vi "功能码解析.vi"(1 "功能码":string) -> ()   [LabVIEW 2013]
panel:
  out "24":bool[](array[boolean])
  out "23":bool[](array[boolean])
  out "22":bool[](array[boolean])
  out "21":bool[](array[boolean])
  out "20":bool[](array[boolean])
  out "19":bool[](array[boolean])
  out "18":bool[](array[boolean])
  out "17":bool[](array[boolean])
  out "16":bool[](array[boolean])
  out "15":bool[](array[boolean])
  out "14":bool[](array[boolean])
  out "13":bool[](array[boolean])
  out "12":bool[](array[boolean])
  out "主板控制类信息10":bool[](array[boolean])
  out "主板版本号11":bool[](array[boolean])
  out "主板故障阀值8":bool[](array[boolean])
  out "主板故障阀值9":bool[](array[boolean])
  out "主板项目信息7":bool[](array[boolean])
  out "主板项目信息6":bool[](array[boolean])
  out "主板项目信息5":bool[](array[boolean])
  out "主板项目信息4":bool[](array[boolean])
  out "主板项目信息3":bool[](array[boolean])
  out "主板监控2":bool[](array[boolean])
  out "主板监控预留1":bool[](array[boolean])
  # "从左到右，从高到低"
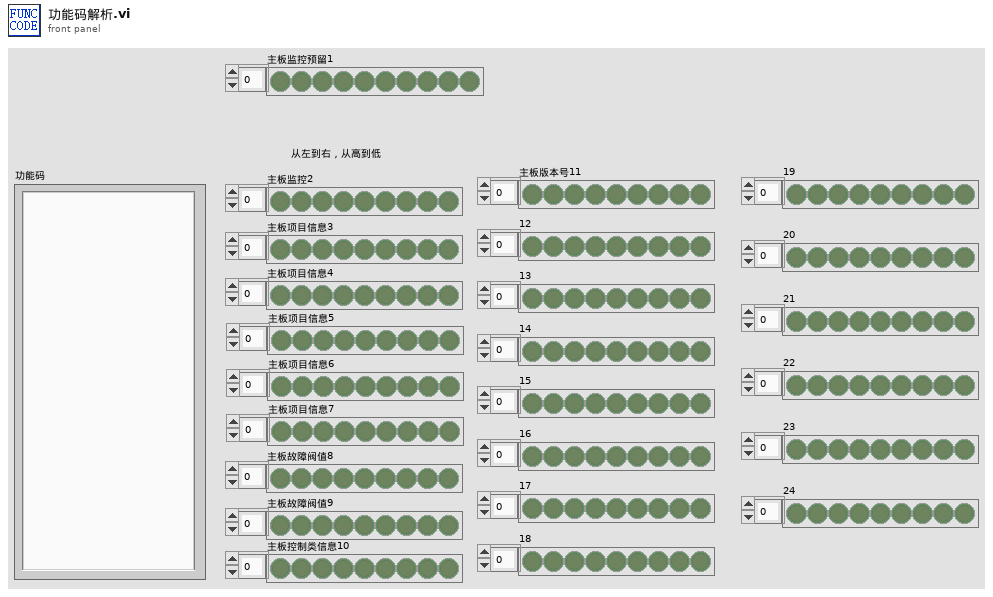
[diagram p1: front panel]
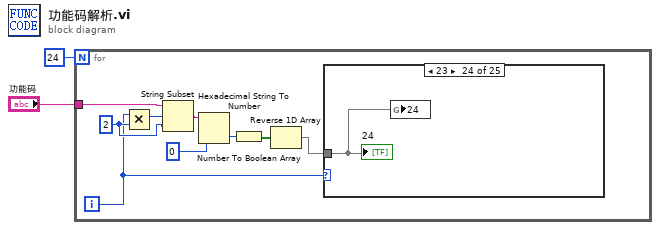
[diagram p0: block diagram]
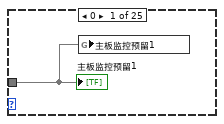
[diagram p2: hidden frame]
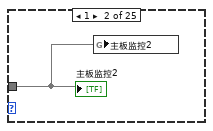
[diagram p3: hidden frame]
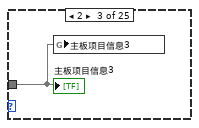
[diagram p4: hidden frame]
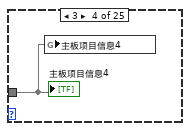
[diagram p5: hidden frame]
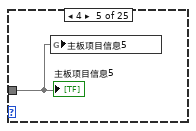
[diagram p6: hidden frame]
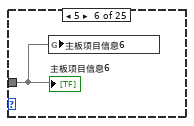
[diagram p7: hidden frame]
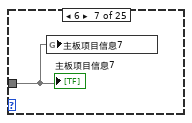
[diagram p8: hidden frame]
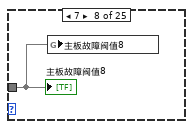
[diagram p9: hidden frame]
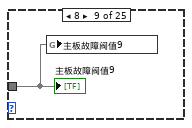
[diagram p10: hidden frame]
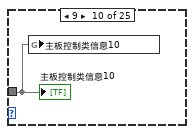
[diagram p11: hidden frame]
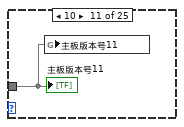
[diagram p12: hidden frame]
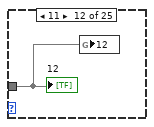
[diagram p13: hidden frame]
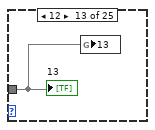
[diagram p14: hidden frame]
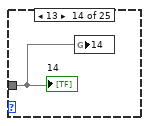
[diagram p15: hidden frame]
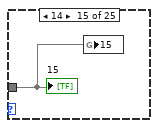
[diagram p16: hidden frame]
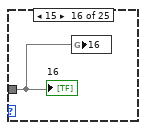
[diagram p17: hidden frame]
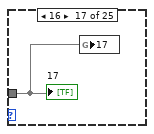
[diagram p18: hidden frame]
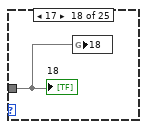
[diagram p19: hidden frame]
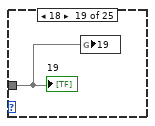
[diagram p20: hidden frame]
diagram:
  n1 = for {
    N: 24 -> [_]
    tunnel: "功能码" -> [w10]
    i -> [w4]
    w9 = 2 ("y")
    n2 = Multiply(x=w4, y=w9) -> (x*y=w11:i32)
    n3 = String Subset(string=w10, offset (0)=w11, length (rest)=w9) -> (substring=w5:string)
    n4 = Hexadecimal String To Number(string=w5, default (0uL)=u8 0) -> (number=w6:u8)  [unwired: 1 in, 1 out]
    n5 = Number To Boolean Array(number=w6) -> (Boolean array=w7:bool[])
    n6 = Reverse 1D Array(array=w7) -> (reversed array=w3:bool[])
    n7 = case shown="23" w4 {
      tunnel: w3 -> [w12 w13 w14 w15 w16 w17 w18 w19 w20 w21 w22 w23 w24 w25 w26 w27 w28 w29 w30 w31 w32 w33 w34 w35 _]
      frame 0 {
        n8 = global write "功能码全局.vi" "主板监控预留1"(w12) -> ()
        "主板监控预留1" <- w12
      }
      frame 1 {
        n9 = global write "功能码全局.vi" "主板监控2"(w13) -> ()
        "主板监控2" <- w13
      }
      frame 2 {
        n10 = global write "功能码全局.vi" "主板项目信息3"(w14) -> ()
        "主板项目信息3" <- w14
      }
      frame 3 {
        n11 = global write "功能码全局.vi" "主板项目信息4"(w15) -> ()
        "主板项目信息4" <- w15
      }
      frame 4 {
        n12 = global write "功能码全局.vi" "主板项目信息5"(w16) -> ()
        "主板项目信息5" <- w16
      }
      frame 5 {
        n13 = global write "功能码全局.vi" "主板项目信息6"(w17) -> ()
        "主板项目信息6" <- w17
      }
      frame 6 {
        n14 = global write "功能码全局.vi" "主板项目信息7"(w18) -> ()
        "主板项目信息7" <- w18
      }
      frame 7 {
        n15 = global write "功能码全局.vi" "主板故障阀值8"(w19) -> ()
        "主板故障阀值8" <- w19
      }
      frame 8 {
        n16 = global write "功能码全局.vi" "主板故障阀值9"(w20) -> ()
        "主板故障阀值9" <- w20
      }
      frame 9 {
        n17 = global write "功能码全局.vi" "主板控制类信息10"(w21) -> ()
        "主板控制类信息10" <- w21
      }
      frame 10 {
        n18 = global write "功能码全局.vi" "主板版本号11"(w22) -> ()
        "主板版本号11" <- w22
      }
      frame 11 {
        n19 = global write "功能码全局.vi" "12"(w23) -> ()
        "12" <- w23
      }
      frame 12 {
        n20 = global write "功能码全局.vi" "13"(w24) -> ()
        "13" <- w24
      }
      frame 13 {
        n21 = global write "功能码全局.vi" "14"(w25) -> ()
        "14" <- w25
      }
      frame 14 {
        n22 = global write "功能码全局.vi" "15"(w26) -> ()
        "15" <- w26
      }
      frame 15 {
        n23 = global write "功能码全局.vi" "16"(w27) -> ()
        "16" <- w27
      }
      frame 16 {
        n24 = global write "功能码全局.vi" "17"(w28) -> ()
        "17" <- w28
      }
      frame 17 {
        n25 = global write "功能码全局.vi" "18"(w29) -> ()
        "18" <- w29
      }
      frame 18 {
        n26 = global write "功能码全局.vi" "19"(w30) -> ()
        "19" <- w30
      }
      frame 19 {
        n27 = global write "功能码全局.vi" "20"(w31) -> ()
        "20" <- w31
      }
      frame 20 {
        n28 = global write "功能码全局.vi" "21"(w32) -> ()
        "21" <- w32
      }
      frame 21 {
        n29 = global write "功能码全局.vi" "22"(w33) -> ()
        "22" <- w33
      }
      frame 22 {
        n30 = global write "功能码全局.vi" "23"(w34) -> ()
        "23" <- w34
      }
      frame 23 {
        n31 = global write "功能码全局.vi" "24"(w35) -> ()
        "24" <- w35
      }
      frame 99, Default {
      }
    }
  }
